vi "Error.vi"(8 "Error":T1) -> (0 "error cluster":errorcluster)   [LabVIEW 2011, in "Tinkerforge.lvlib" / "IP Connection.lvclass"]
doc: "This VI returns the <B>Error Cluster</B> to the given <B>Error</B>."
uses:
  IP Connection.lvclass
  Type Definitions/Errors.ctl
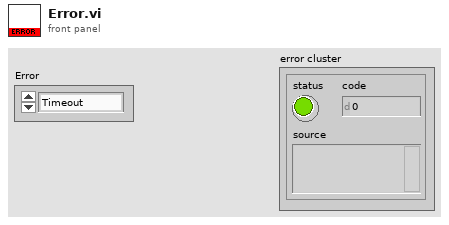
[diagram p1: front panel]
types:
  T1 = typedef "Tinkerforge.lvlib/IP Connection.lvclass/Errors.ctl" = enum16{"Timeout", "Device type incorrect", "Device already added", "Device not existing"}
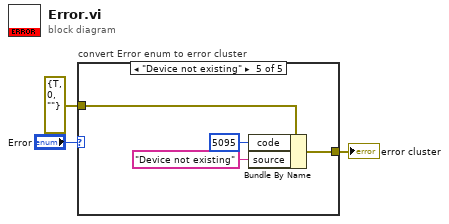
[diagram p0: block diagram]
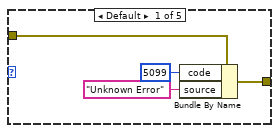
[diagram p2: hidden frame]
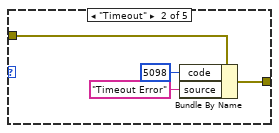
[diagram p3: hidden frame]
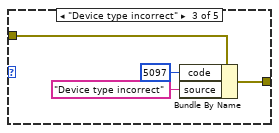
[diagram p4: hidden frame]
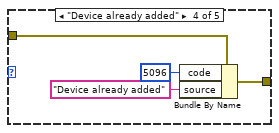
[diagram p5: hidden frame]
diagram:
  n1 = case "convert Error enum to error cluster" shown="\"Device not existing\"" "Error" {
    tunnel: errorcluster {"status"=TRUE, "code"=0, "source"=""} ("error constant") -> [w7 w11 w15 w19 w23]
    tunnel: [w4 w8 w12 w16 w20] -> w1
    frame Default {
      n2 = Bundle By Name(cluster=w7, "code"=5099, "source"="Unknown Error") -> (w4:errorcluster)
    }
    frame "Timeout" {
      n3 = Bundle By Name(cluster=w11, "code"=5098, "source"="Timeout Error") -> (w8:errorcluster)
    }
    frame "Device type incorrect" {
      n4 = Bundle By Name(cluster=w15, "code"=5097, "source"="Device type incorrect") -> (w12:errorcluster)
    }
    frame "Device already added" {
      n5 = Bundle By Name(cluster=w19, "code"=5096, "source"="Device already added") -> (w16:errorcluster)
    }
    frame "Device not existing" {
      n6 = Bundle By Name(cluster=w23, "code"=5095, "source"="Device not existing") -> (w20:errorcluster)
    }
  }
  "error cluster" <- w1
